vi "Robot Global Data.vi"() -> ()   [LabVIEW 2019]
doc: "This global VI can contain as many global variables as you need. Place a control on the panel, give it a good name. To read or write to it from a VI, drag the icon to the diagram of that VI. You can also drag from the project. Click on the node to change which global you access. You shouldn't have multiple locations writing to a global or it will cause a race-condition."
uses:
  <vilib>/Rock Robotics/WPI/Camera/WPI_CameraImageSize.ctl
  <vilib>/Rock Robotics/WPI/DriverStation/WPI_DriverStationRobotMode2.ctl
panel:
  out "DiffDrSim_RMotDmd":dbl format="%17.2f"
  out "DiffDrSim_LMotDmd":dbl format="%17.2f"
  out "DiffDrSim_DriveCurrent":dbl format="%17.2f"
  out "DiffDrSim_BattVolts":dbl format="%17.2f"
  out "DiffDrSim_Heading":dbl format="%17.2f"
  out "DiffDrSim_RPos":dbl format="%17.2f"
  out "DiffDrSim_LPos":dbl format="%17.2f"
  out "DiffDrSim_RVel":dbl format="%17.2f"
  out "DiffDrSim_LVel":dbl format="%17.2f"
  out "Traj Samp Pose Y":dbl format="%17.2f"
  out "Traj Samp Pose X":dbl format="%17.2f"
  out "Traj Samp Curvature":dbl format="%17.2f"
  out "Traj Samp Accel":dbl format="%17.2f"
  out "Traj Samp Velocity":dbl format="%17.2f"
  out "Traj Samp Time":dbl format="%17.2f"
  out "Traj_RamseteEnabled":bool
  out "Traj Y CorrXX":dbl format="%17.2f"
  out "Traj X CorrXX":dbl format="%17.2f"
  out "Traj Closed LoopXX":bool
  out "Traj Curvature SampleXX":dbl format="%17.2f"
  out "Traj Velocity SampleXX":dbl format="%17.2f"
  out "Traj Heading SampleXX":dbl format="%17.2f"
  out "Traj Y SampleXX":dbl format="%17.2f"
  out "Traj X SampleXX":dbl format="%17.2f"
  out "Traj_IsGood":bool
  out "Traj_Total_Time":dbl format="%17.2f"
  out "Traj_Total_States":dbl format="%17.2f"
  out "Traj Heading Err":dbl format="%17.2f"
  out "Traj Y Err":dbl format="%17.2f"
  out "Traj X Err":dbl format="%17.2f"
  out "Traj_OnTarget":bool
  out "GyroCont":dbl format="%17.2f"
  out "DrvDistCalcLeftTest":dbl format="%17.2f"
  out "DrvDistCalcRightTest":dbl format="%17.2f"
  out "DrvDistReadLeft":dbl format="%17.2f"
  out "DrvDistReadRight":dbl format="%17.2f"
  out "DrvSpeedLeft":dbl format="%17.2f"
  out "DrvSpeedRight":dbl format="%17.2f"
  out "DrvMotorOutLeft":dbl format="%17.2f"
  out "DrvMotorOutRight":dbl format="%17.2f"
  out "DrvSpeedDmdLeft":dbl format="%17.2f"
  out "DrvSpeedDmdRight":dbl format="%17.2f"
  out "DrvSpeedTargLeft":dbl format="%17.2f"
  out "DrvSpeedTargRight":dbl format="%17.2f"
  in  "Robot Mode":T1
  in  "image size":T2=enum."320x240"
  in  "Enable Vision":bool
  # "DIFF DRIVE TRAIN SIM"
  # "Left over from diferential drive!!"
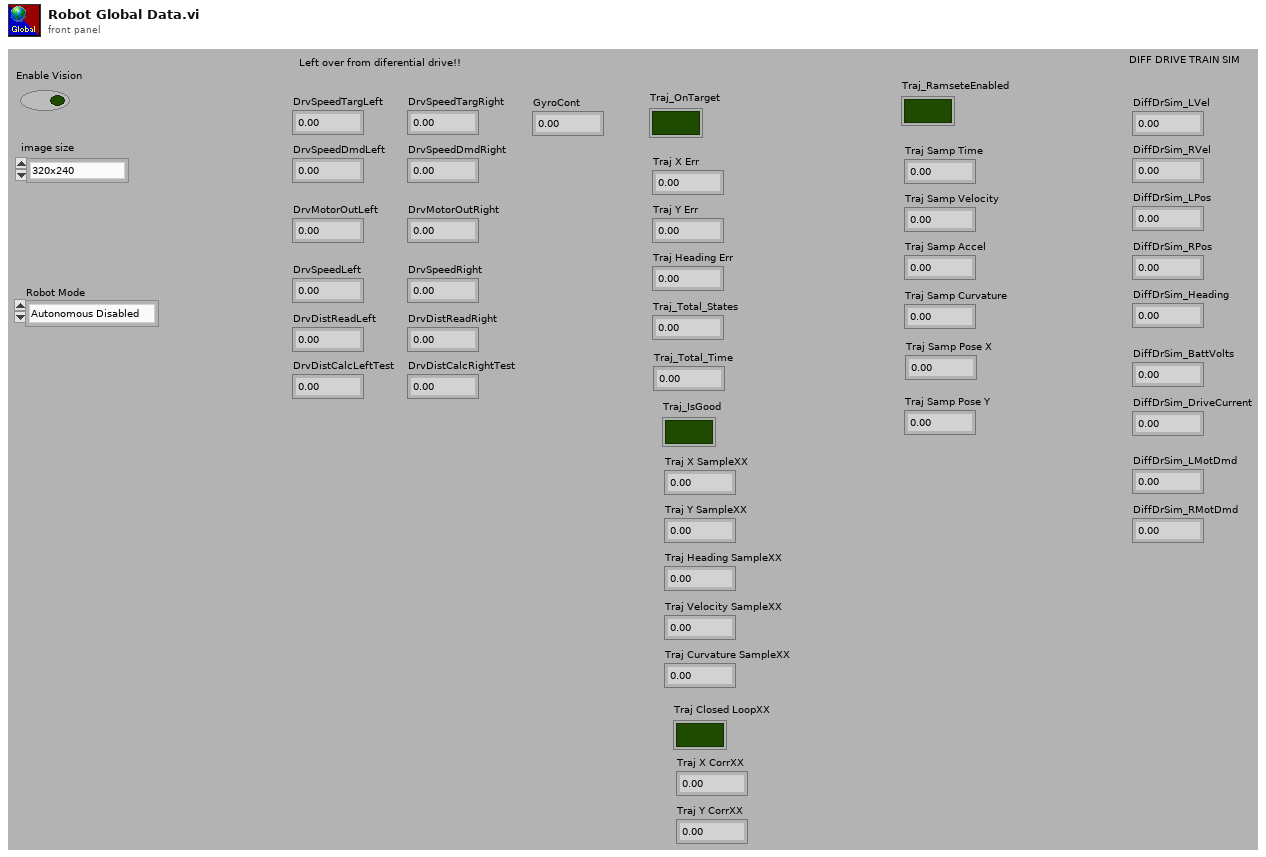
[diagram p1: front panel]
types:
  T1 = typedef "WPI_DriverStationRobotMode2.ctl" = enum16{"Autonomous Disabled", "Autonomous Enabled", "Teleop Disabled", "Teleop Enabled", "Disconnected", "Finish", "Test Disabled", "Test Enabled", "Emergency Stopped"}
  T2 = typedef "WPI_CameraImageSize.ctl" = enum16{"640x480", "320x240", "160x120", "Custom"}
diagram:
